vi "Calibrate VNA Dialog.vi"(8 "error in (no error)":errorcluster, 11 "Vector Network Analyzer in":refnum<class "Vector Network Analyzer.lvclass">) -> (0 "error out":errorcluster, 3 "Vector Network Analyzer out":refnum<class "Vector Network Analyzer.lvclass">)   [LabVIEW 2020, in "Vector Network Analyzer.lvclass"]
doc: "Calibration of the VNA.\nThis is a dialog interface for the user to setup the VNA prior to calibration."
uses:
  Vector Network Analyzer.lvclass
  Controls/S parm format enum.ctl
  Vector Network Analyzer.lvclass/Vector Network Analyzer.ctl
panel:
  in  "Power [dBm]":dbl
  in  "Calibration mode":u16(ring)=1 items=["1 Port", "2 Port", "3 Port", "4 Port"]
  in  "Calibration Kit":u16(ring) items=["E-CAL", "3.5 mm Ideal Kit", "3650-1", "85052D", "Maury 8050", "ZV-Z132", "ZV-Z135 typical", "ZV-Z32 typical", "ZV-Z33 typical", "85033D/E", "85052B", "85052C", "ZV-Z135"]
  in  "Average On":bool
  in  "Averages":i32
  in  "Run Cal Button":bool
  in  "Number of Points":i32
  in  "IF BW":dbl format="%#_6p"
  in  "Stop Frequency":dbl format="%#_6p"
  in  "Start Frequency":dbl format="%#_6p"
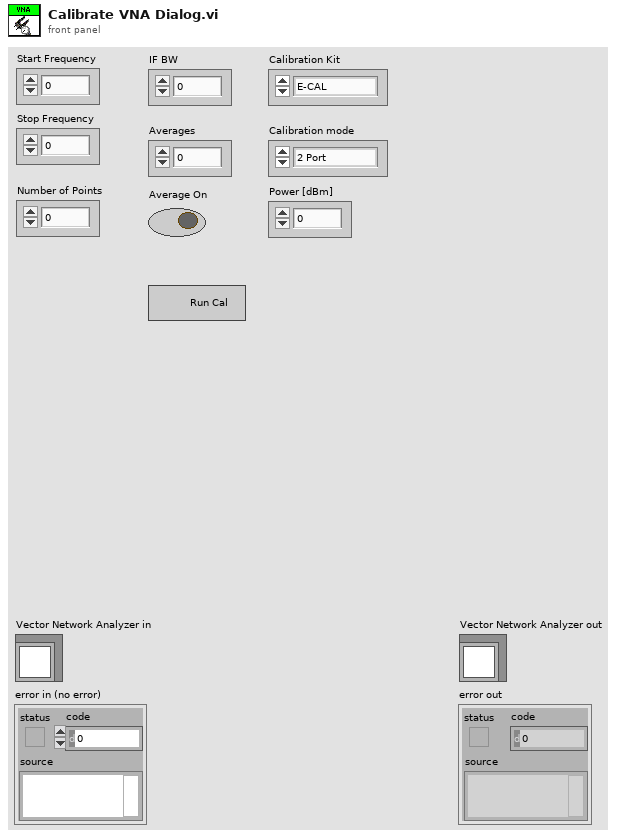
[diagram p1: front panel]
types:
  T1 = typedef "Vector Network Analyzer.lvclass/S parm format enum.ctl" = enum16{"Mag dB", "Mag", "Phase", "Smith", "Real", "Imag", "Group Delay", "SWR"}
  T2 = enum16{"S11", "S21", "S31", "S41", "S22", "S12", "S32", "S42", "S33", "S13", "S23", "S43", "S44", "S14", "S24", "S34"}
  T3 = enum16{"SMA/3.5 mm", "2.92 mm", "2.4 mm", "1.85 mm", "N 50 Ohm", "N 75 Ohm", "7-16"}
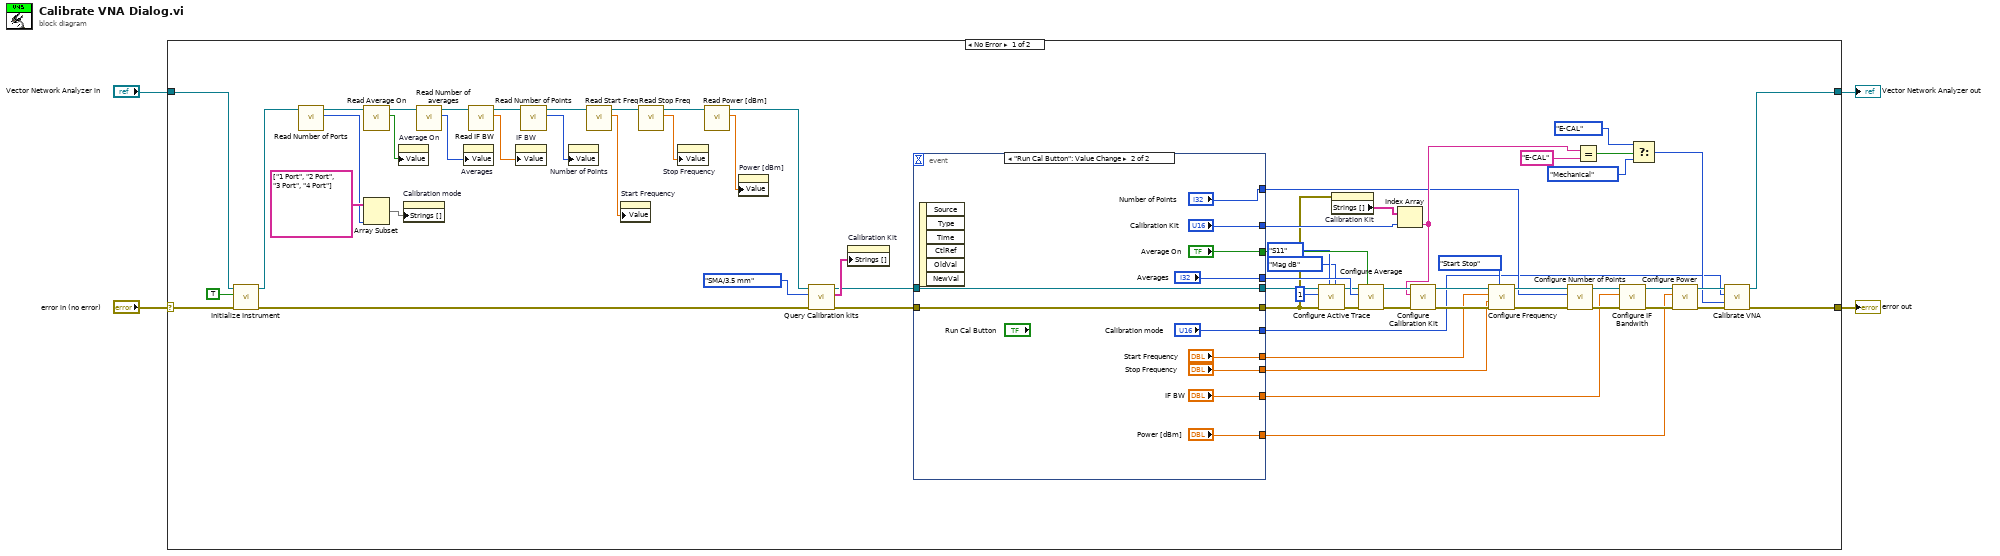
[diagram p0: block diagram]
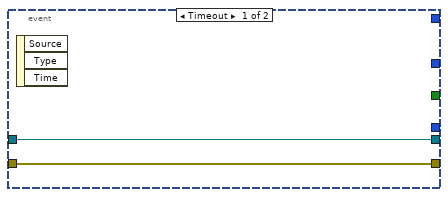
[diagram p2: hidden frame]
diagram:
  n1 = case shown="No Error" "error in (no error)" {
    selector: "error in (no error)" -> [w69 w84]
    tunnel: [w22 w84] -> w3
    tunnel: [w21 w83] -> w1
    tunnel: "Vector Network Analyzer in" -> [w68 w83]
    frame No Error {
      n2 = call-dynamic "Initialize Instrument.vi"("error in (no error)"=w69, "Reset"=TRUE, "Instrument in"=w68) -> ("error out"=w50:errorcluster, "Instrument out"=w66:refnum<class "Vector Network Analyzer.lvclass">)  [unwired: 7 in]
      n3 = call "Read Number of Ports.vi"("Vector Network Analyzer in"=w66) -> ("Number of Ports"=w59:i32, "Vector Network Analyzer out"=w65:refnum<class "Vector Network Analyzer.lvclass">)  [unwired: 9 in]
      n4 = call "Read Average On.vi"("Vector Network Analyzer in"=w65) -> ("Average On"=w64:bool, "Vector Network Analyzer out"=w63:refnum<class "Vector Network Analyzer.lvclass">)  [unwired: 9 in]
      n5 = Array Subset(array=string[] ["1 Port", "2 Port", "3 Port", "4 Port"], length=w59) -> (w58:string[])  [unwired: 1 in]
      n6 = property on="Average On" class="Bool (strict)"("Value"=w64) -> ()  [unwired: 2 in, 2 out]
      n7 = property on="Calibration mode" class="Ring (strict)"("Strings []"=w58) -> ()  [unwired: 2 in, 2 out]
      n8 = call "Read Number of averages.vi"("Vector Network Analyzer in"=w63) -> ("Number of averages"=w62:i32, "Vector Network Analyzer out"=w61:refnum<class "Vector Network Analyzer.lvclass">)  [unwired: 9 in]
      n9 = property on="Averages" class="DigNum (strict)"("Value"=w62) -> ()  [unwired: 2 in, 2 out]
      n10 = call "Read IF BW.vi"("Vector Network Analyzer in"=w61) -> ("IF BW"=w57:dbl, "Vector Network Analyzer out"=w56:refnum<class "Vector Network Analyzer.lvclass">)  [unwired: 9 in]
      n11 = property on="IF BW" class="DigNum (strict)"("Value"=w57) -> ()  [unwired: 2 in, 2 out]
      n12 = call "Read Number of Points.vi"("Vector Network Analyzer in"=w56) -> ("Number of Points"=w55:i32, "Vector Network Analyzer out"=w54:refnum<class "Vector Network Analyzer.lvclass">)  [unwired: 9 in]
      n13 = property on="Number of Points" class="DigNum (strict)"("Value"=w55) -> ()  [unwired: 2 in, 2 out]
      n14 = call "Read Start Freq.vi"("Vector Network Analyzer in"=w54) -> ("Start Freq"=w52:dbl, "Vector Network Analyzer out"=w53:refnum<class "Vector Network Analyzer.lvclass">)  [unwired: 9 in]
      n15 = property on="Start Frequency" class="DigNum (strict)"("Value"=w52) -> ()  [unwired: 2 in, 2 out]
      n16 = call "Read Stop Freq.vi"("Vector Network Analyzer in"=w53) -> ("Stop Freq"=w51:dbl, "Vector Network Analyzer out"=w37:refnum<class "Vector Network Analyzer.lvclass">)  [unwired: 9 in]
      n17 = property on="Stop Frequency" class="DigNum (strict)"("Value"=w51) -> ()  [unwired: 2 in, 2 out]
      n18 = call "Read Power [dBm].vi"("Vector Network Analyzer in"=w37) -> ("Power [dBm]"=w35:dbl, "Vector Network Analyzer out"=w36:refnum<class "Vector Network Analyzer.lvclass">)  [unwired: 9 in]
      n19 = property on="Power [dBm]" class="DigNum (strict)"("Value"=w35) -> ()  [unwired: 2 in, 2 out]
      n20 = call-dynamic "Query Calibration kits.vi"("error in (no error)"=w50, "Connector type"=T3."SMA/3.5 mm", "Vector Network Analyzer in"=w36) -> ("error out"=w47:errorcluster, "Cal kits installed"=w48:string[], "Vector Network Analyzer out"=w46:refnum<class "Vector Network Analyzer.lvclass">)  [unwired: 6 in]
      n21 = property on="Calibration Kit" class="Ring (strict)"("Strings []"=w48) -> ()  [unwired: 2 in, 2 out]
      n22 = event shown="[1] \"Run Cal Button\": Value Change" {
        selector: _ -> [_ _]
        dyn-events: _ -> [_ _]
        timeout: _ -> [_ _]
        tunnel: w47 -> [w70 w81]
        tunnel: w46 -> [w71 w82]
        tunnel: [w71 w82] -> w9
        tunnel: [w70 w81] -> w8
        tunnel: [_ "Calibration Kit"] -> w20
        tunnel: [_ "Averages"] -> w19
        tunnel: [_ "Average On"] -> w18
        tunnel: [_ "Number of Points"] -> w17
        tunnel: [_ "Calibration mode"] -> w16
        tunnel: [_ "Start Frequency"] -> w15
        tunnel: [_ "Stop Frequency"] -> w14
        tunnel: [_ "IF BW"] -> w13
        tunnel: [_ "Power [dBm]"] -> w12
        event Timeout {
          n23 = event-data() -> ()  [unwired: 1 in, 3 out]
        }
        event "Run Cal Button": Value Change {
          n24 = event-data() -> ()  [unwired: 1 in, 6 out]
        }
      }
      n25 = call-dynamic "Configure Active Trace.vi"("Format"=S_parm_format_enum."Mag dB", "S parameter"=T2."S11", "error in (no error)"=w8, "Active Trace"=u8 1, "Vector Network Analyzer in"=w9) -> ("error out"=w11:errorcluster, "Vector Network Analyzer out"=w10:refnum<class "Vector Network Analyzer.lvclass">)  [unwired: 5 in]
      n26 = property on="Calibration Kit" class="Ring (strict)"(error in=w8) -> ("Strings []"=w44:string[])  [unwired: 1 in, 2 out]
      n27 = call-dynamic "Configure Average.vi"("Average On"=w18, "error in (no error)"=w11, "Number of Averages"=w19, "Vector Network Analyzer in"=w10) -> ("error out"=w43:errorcluster, "Vector Network Analyzer out"=w45:refnum<class "Vector Network Analyzer.lvclass">)  [unwired: 6 in]
      n28 = Index Array(array=w44, index=w20) -> (element=w28:string)
      n29 = call-dynamic "Configure Calibration Kit.vi"("error in (no error)"=w43, "Cal kit Name"=w28, "Vector Network Analyzer in"=w45) -> ("error out"=w42:errorcluster, "Vector Network Analyzer out"=w41:refnum<class "Vector Network Analyzer.lvclass">)  [unwired: 7 in]
      n30 = call-dynamic "Configure Frequency.vi"("Mode"=enum16{"Center Span", "Start Stop"}."Start Stop", "error in (no error)"=w42, "Span/Stop Frequency"=w14, "Center/Start Frequency"=w15, "Vector Network Analyzer in"=w41) -> ("error out"=w39:errorcluster, "Vector Network Analyzer out"=w38:refnum<class "Vector Network Analyzer.lvclass">)  [unwired: 5 in]
      n31 = call-dynamic "Configure Number of Points.vi"("error in (no error)"=w39, "Number of Point"=w17, "Vector Network Analyzer in"=w38) -> ("error out"=w34:errorcluster, "Vector Network Analyzer out"=w33:refnum<class "Vector Network Analyzer.lvclass">)  [unwired: 7 in]
      n32 = Equal?(x=w28, y="E-CAL") -> (x = y?=w26:bool)
      n33 = call-dynamic "Configure IF Bandwith.vi"("error in (no error)"=w34, "IF BW [Hz]"=w13, "Vector Network Analyzer in"=w33) -> ("error out"=w32:errorcluster, "Vector Network Analyzer out"=w31:refnum<class "Vector Network Analyzer.lvclass">)  [unwired: 6 in, 1 out]
      n34 = Select(t=enum16{"E-CAL", "Mechanical"}."E-CAL" ("Cal kit type"), s=w26, f=enum16{"E-CAL", "Mechanical"}."Mechanical") -> (s? t:f=w23:enum16{"E-CAL", "Mechanical"})
      n35 = call-dynamic "Configure Power.vi"("error in (no error)"=w32, "Power [dBm]"=w12, "Vector Network Analyzer in"=w31) -> ("error out"=w30:errorcluster, "Vector Network Analyzer out"=w29:refnum<class "Vector Network Analyzer.lvclass">)  [unwired: 7 in]
      n36 = call-dynamic "Calibrate VNA.vi"("error in (no error)"=w30, "Cal kit type"=w23, "Calibration mode"=w16, "Vector Network Analyzer in"=w29) -> ("error out"=w22:errorcluster, "Vector Network Analyzer out"=w21:refnum<class "Vector Network Analyzer.lvclass">)  [unwired: 6 in]
    }
    frame Error {
    }
  }
  "error out" <- w3
  "Vector Network Analyzer out" <- w1
